vi "CRYGet Date Time.vi"() -> (0 "time":string, 3 "date":string)   [LabVIEW 2013]
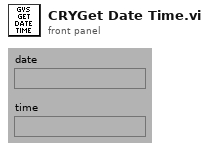
[diagram p1: front panel]
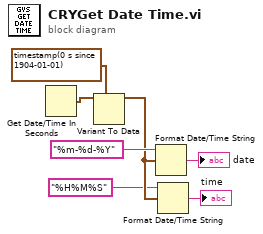
[diagram p0: block diagram]
diagram:
  n1 = Get Date/Time In Seconds() -> (seconds since 1Jan1904=w7:timestamp)
  n2 = Variant To Data(type=timestamp(0 s since 1904-01-01) ("Time Stamp"), Variant=w7) -> (data=w3:timestamp)  [unwired: 1 in, 1 out]
  n3 = Format Date/Time String(time format string (%c)="%m-%d-%Y", seconds (now)=w3) -> (date/time string=→"date":string)  [unwired: 1 in]
  n4 = Format Date/Time String(time format string (%c)="%H%M%S", seconds (now)=w3) -> (date/time string=→"time":string)  [unwired: 1 in]
